vi "doESR.vi"(6 "IntGraph Refnum":refnum<vi>, 8 "current_run_ref":refnum<vi>, 9 "generator_enable":bool, 10 "sweep_parameters":T1={"Repetitions"=1, "Power dBm"=5.999999061226845, "Freq Start [Hz]"=2800000000.0, "Freq Stop [Hz]"=3000000000.0, "Step size [Hz]"=2500000.0, "Dwell Time [s]"=0.09999999974525053} {"Dwell Time [s]" format="%.3f"; "Step size [Hz]" format="%.2p"; "Freq Stop [Hz]" format="%.2p"; "Freq Start [Hz]" format="%.2p"; "Power dBm" format="%.2f"; "Repetitions" min=1 max=1000 step=1}, 11 "position_xyz":T2 {"Position Z" min=0.0 max=10.0 step=0.001 format="%.3f"; "Position Y" min=-10.0 max=10.0 step=0.1 format="%.3f"; "Position X" min=-10.0 max=10.0 step=0.1 format="%.3f"}) -> ()   [LabVIEW 2014]
uses:
  GLOBAL_VAR.vi
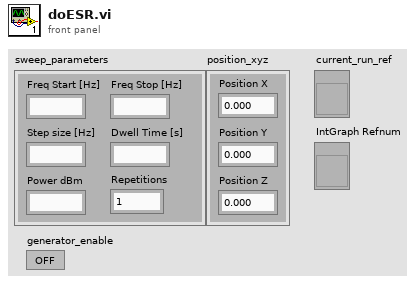
[diagram p1: front panel]
types:
  T1 = cluster{"Repetitions":i32, "Power dBm":ext, "Freq Start [Hz]":ext, "Freq Stop [Hz]":ext, "Step size [Hz]":ext, "Dwell Time [s]":ext}
  T2 = cluster{"Position X":dbl, "Position Y":dbl, "Position Z":dbl}
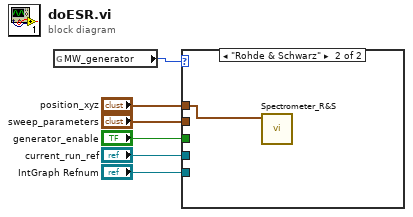
[diagram p0: block diagram]
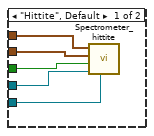
[diagram p2: hidden frame]
diagram:
  n1 = global read "GLOBAL_VAR.vi" "MW_generator"() -> (w6:enum32{"Hittite", "Rohde & Schwarz"})
  n2 = case shown="\"Rohde & Schwarz\"" w6 {
    tunnel: "position_xyz" -> [w11 w12]
    tunnel: "sweep_parameters" -> [w10 _]
    tunnel: "generator_enable" -> [w9 _]
    tunnel: "current_run_ref" -> [w8 _]
    tunnel: "IntGraph Refnum" -> [w7 _]
    frame "Hittite", Default {
      n3 = call "Spectrometer_hittite.vi"("ESR_stack_ref"=w7, "current_run_ref"=w8, "generator_enable"=w9, "sweep_parameters"=w10, "position_xyz"=w11) -> ()  [unwired: 7 in]
    }
    frame "Rohde & Schwarz" {
      n4 = call "Spectrometer_R&S.vi"("position_xyz"=w12) -> ()  [unwired: 11 in]
    }
  }
